vi "ReadPowerSetting(General).vi"(8 "Error In":errorcluster, 11 "VISA resource name":refnum<visa-resource-name>) -> (0 "Error Out":errorcluster, 2 "Setting":dbl, 3 "VISA resource name out":refnum<visa-resource-name>)   [LabVIEW 2013]
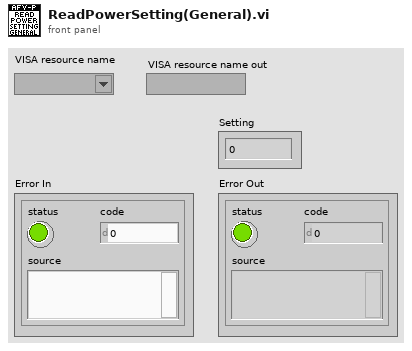
[diagram p1: front panel]
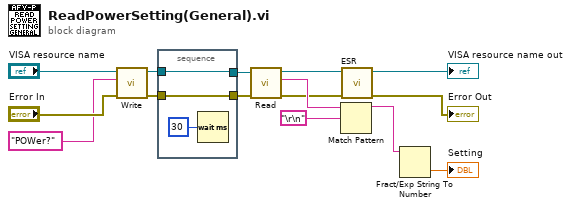
[diagram p0: block diagram]
diagram:
  n1 = call "Write.vi"("Error In"="Error In", "Write Buffer"="POWer?", "VISA resource name"="VISA resource name") -> ("Error Out"=w10:errorcluster, "VISA resource name out"=w13:refnum<visa-resource-name>)  [unwired: 7 in]
  n2 = stacked-sequence {
    tunnel: [w17] -> w12
    tunnel: w13 -> [w17]
    tunnel: [w16] -> w11
    tunnel: w10 -> [w16]
    frame #0 {
      n3 = Wait (ms)(milliseconds to wait=u32 30) -> ()  [unwired: 1 out]
    }
  }
  n4 = call "Read.vi"("Error In"=w11, "VISA resource name"=w12) -> ("Error Out"=w8:errorcluster, "Read Data"=w9:string, "VISA resource name out"=w7:refnum<visa-resource-name>)  [unwired: 7 in]
  n5 = Match Pattern(string=w9, regular expression="\r\n") -> (before substring=w1:string)  [unwired: 1 in, 3 out]
  n6 = call "ESR.vi"("Error In"=w8, "VISA resource name"=w7) -> ("Error Out"=→"Error Out":errorcluster, "VISA resource name out"=→"VISA resource name out":refnum<visa-resource-name>)  [unwired: 8 in]
  n7 = Fract/Exp String To Number(string=w1) -> (number=→"Setting":dbl)  [unwired: 3 in, 1 out]
